vi "XMLdoublequote.vi"(8 "error in (no error)":errorcluster, 10 "XML Input":string) -> (0 "error out":errorcluster, 2 "XML Output":string)   [LabVIEW 2014]
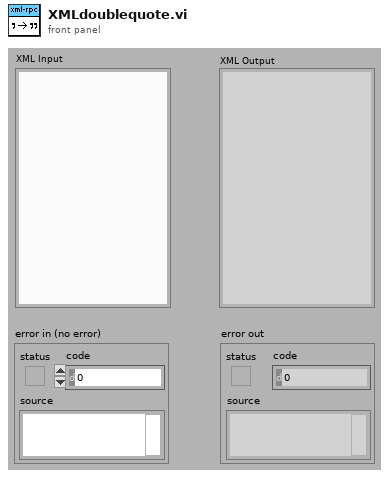
[diagram p1: front panel]
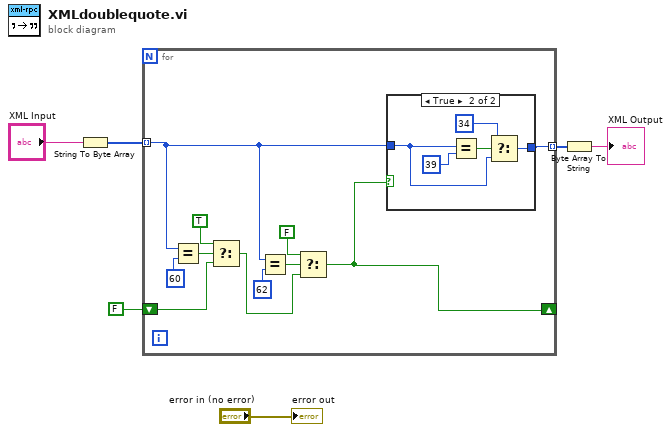
[diagram p0: block diagram]
diagram:
  n1 = String To Byte Array(string="XML Input") -> (unsigned byte array=w5:u8[])
  n2 = for {
    tunnel: w5 -> [w10] mode=indexing
    tunnel: [w17] -> w4 mode=indexing
    shift-right: [w7] -> _
    shift-left: FALSE -> [w13]
    n3 = Equal?(x=w10, y=u8 60) -> (x = y?=w16:bool)
    n4 = Select(t=TRUE, s=w16, f=w13) -> (s? t:f=w8:bool)
    n5 = Equal?(x=w10, y=u8 62) -> (x = y?=w12:bool)
    n6 = Select(t=FALSE, s=w12, f=w8) -> (s? t:f=w7:bool)
    n7 = case shown="True" w7 {
      tunnel: w10 -> [w18 w20]
      tunnel: [w18 w19] -> w17
      frame False {
      }
      frame True {
        n8 = Equal?(x=w20, y=u8 39) -> (x = y?=w22:bool)
        n9 = Select(t=i8 34, s=w22, f=w20) -> (s? t:f=w19:u8)
      }
    }
  }
  n10 = Byte Array To String(unsigned byte array=w4) -> (string=→"XML Output":string)
  "error out" <- "error in (no error)"
